vi "04control logicas slave.vi"(4 "COM DATA":T1, 5 "DATO":u32, 7 "Equipo Nº":u8) -> (1 "error out":errorcluster)   [LabVIEW 2010]
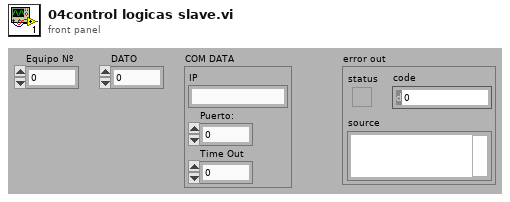
[diagram p1: front panel]
types:
  T1 = cluster{"IP ":string, "Puerto:":u16, "Time Out":u16}
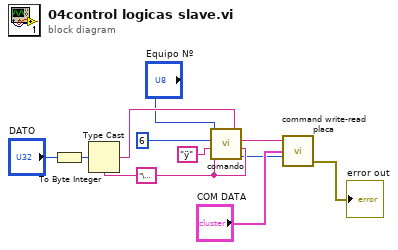
[diagram p0: block diagram]
diagram:
  w7 = "\u0000" ("LOW")
  n1 = To Byte Integer(number="DATO") -> (8bit integer=w1:i8)
  n2 = Type Cast(type=w7, x=w1) -> (*(type *) &x=w10:string)
  n3 = call "comando.vi"("ANEXO L"=w7, "ANEXO H"=w10, "LOW"=w7, "HIGH"="ÿ" ("ANEXO H"), "Comando:"=u8 6, "Equipo Nº"="Equipo Nº") -> ("Bytes OUT"=w5:u16, "comando"=w4:string)  [unwired: 1 in]
  n4 = call "command write-read placa.vi"("Write Command"=w4, "COM DATA"="COM DATA", "bytes"=w5) -> ("error out"=→"error out":errorcluster)  [unwired: 3 in, 1 out]
